vi "Generate 2D scan Waveform.vi"(8 "error in (no error)":errorcluster, 11 "System Parameters [In]":T1={"Optical Parameters"={"Obj. Focal Length [mm]"=0.0, "Scan Lens EFL[mm]"=0.0, "Tube Lens EFL[mm]"=0.0, "Galvo V Range (+/-)"=10.0, "Galvo Max Half Angle [Deg]"=18.0, "Max Galvo Range[%]"=90.0}, "Vibratome"={"Z Bottom [mm]"=0.0, "Pre Cut Dwell [s]"=0.0, "Blade Frequency [RPM]"=0, "Slice Speed [mm/s]"=0.0, "Post Cut Dwell [s]"=0.0, "Ramp Time [s]"=0.0, "Start X [mm]"=0.0, "Start Y [mm]"=0.0, "Slice Length [mm]"=0.0, "Slice Axis"=enum."Y Axis", "Controller VISA Ref"="COM4", "Blade Frequency [Hz]"=0, "Analog Out Channel"="GalvoCtrl/ao0,GalvoCtrl/ao1", "Pixel Clock Source"="/GalvoCtrl/PFI0"}, "Table Stages"={"X Stage"={"Position"=0.0, "Is.Enabled?"=FALSE, "Is.Connected?"=FALSE, "Device SN"="45876539", "AccelerationMaximum"=0.0, "VelocityMaximum"=0.0, "Acceleration"=0.0, "Velocity"=0.0, "waitTimeout (ms)"=0, "Model"=enum."None", "Is.Homed?"=FALSE}, "Y Stage"={"Position"=0.0, "Is.Enabled?"=FALSE, "Is.Connected?"=FALSE, "Device SN"="45876539", "AccelerationMaximum"=0.0, "VelocityMaximum"=0.0, "Acceleration"=0.0, "Velocity"=0.0, "waitTimeout (ms)"=0, "Model"=enum."None", "Is.Homed?"=FALSE}, "Z Stage"={"Position"=0.0, "Is.Enabled?"=FALSE, "Is.Connected?"=FALSE, "Device SN"="45876539", "AccelerationMaximum"=0.0, "VelocityMaximum"=0.0, "Acceleration"=0.0, "Velocity"=0.0, "waitTimeout (ms)"=0, "Model"=enum."None", "Is.Homed?"=FALSE}}, "Imaging Parameter"={"Raster Scan Direction"=enum."Uni Directional", "Pixel Dwell Time [Clock Cycles]"=0, "Flyback Time [Clock Cycles]"=0, "XY Center [um]"={"X"=1.0, "Y"=1.0}, "Pixel Step Size [um] X"=3.0, "XY Image Size"=enum."256 x 256", "Custom"=TRUE, "Custom Size"={"X"=1200, "Y"=1}, "Line Averages"=1, "Pixel Step Size [um] Y"=3.0}, "Galvo HW Parameters"={"Analog Out Channel"="GalvoCtrl/ao0,GalvoCtrl/ao1", "Min Voltage"=-10.0, "Max Voltage"=10.0, "Pixel Clock Source"="/GalvoCtrl/PFI0", "Sample Rate"=1000.0, "Line Clock Out Ch"="GalvoCtrl/port0/line0"}, "Alazar parameters"={"Trigger Settings"={"General Trigger Settings"={"Trigger Operation"=0, "Coupling ID"=2, "Range ID"=2, "Delay"=0, "Timeout Ticks"=0, "Mode"=1, "Parameter"=1}, "Trigger Engine 1"={"Trigger Engine"=0, "Source"=2, "Slope"=1, "Level"=140}, "Trigger Engine 2"={"Trigger Engine"=1000, "Source"=4294967295, "Slope"=1, "Level"=2048}}, "Device ID"={"System ID"=1, "Board ID"=1}, "Ch A Input Control"={"Channel"=1, "Coupling"=2, "Range"=10, "Impedance"=2}, "Ch B Input Control"={"Channel"=2, "Coupling"=2, "Range"=10, "Impedance"=2}, "Acq Settings"={"Record Length"=1440, "Offset"=0, "Records Per Buffer"=2048, "Records Count (Records/Acq)"=2147483647, "Window Type"=1, "Footer"=0, "Samples per record"=2048, "Output Format"=257}, "Capture Clock"={"Sample Rate"=100, "Decimation"=0, "Source"=2, "Edge"=0}}, "Mosaic Paramter"={"X Axis"={"Start [mm]"=0.0, "Steps [pts]"=0.0, "End [mm]"=0.0}, "Y Axis"={"Start [mm]"=0.0, "Steps [pts]"=0.0, "End [mm]"=0.0}, "Scan Pattern"=enum."Uni-directional", "Overlap Options"={"Overlap Type"=enum."No Overlap", "Percent Overlap"=0, "Justify"=enum."Start"}}, "Manual Controls"={"Z0"=10.0, "First image height"=0.0, "Data Path"=path "", "Save parameters"={"start pixel"=45, "#pixels to save"=100}, "Center Galvos"=FALSE, "Acquisition mode"=enum."Alazar FFT", "PSOCT Channel"=1, "Save"=FALSE, "AIP rotation angle"=0.0, "Scan Parameters"={"# Scan"={"#Ascan"=150, "#Bscan"=400}, "# Rpt"={"#ARpt"=1, "#BRpt"=1}, "Aline Rate"=2, "# Extra"={"# ARpt_extra"=5, "#Brtn_extra"=60}}, "ROI Parameters"={"ROI (mm)"={"X (mm)"=1.0, "Y (mm)"=1.0}, "Shift (mm)"={"Xshift (mm)"=0.0, "Yshift (mm)"=0.0}}, "Objective"=30, "ret ds"=FALSE, "Pause?"=FALSE}, "Vibratome Axis"={"Start [mm](first cut height)"=45.85, "slice thickness[um]"=2.1, "#slice"=111, "image thickness(um)"=0.0, "#images"=0, "30um?"=FALSE}} {"Manual Controls"."Objective" items=["5X LKM05", "10X LKM10", "20X LKM20", "10X LSM02"]; "Manual Controls"."Scan Parameters"."Aline Rate" items=["76 KHz", "146 KHz", "76 KHz", "28 KHz", "10 KHz"]; "Manual Controls"."PSOCT Channel" items=["A"=1, "B"=2, "A + B"=3, "C"=4, "A + C"=5, "A + B"=6, "D"=8, "A + D"=9, "B + D"=10, "C + D"=12, "A + B + C + D"=15]; "Alazar parameters"."Capture Clock"."Edge" items=["Rising", "Falling"]; "Alazar parameters"."Capture Clock"."Source" items=["Internal"=1, "Fast External"=2, "Medium External"=3, "Slow External"=4, "External AC"=5, "External DC"=6, "External 10MHz"=7]; "Alazar parameters"."Acq Settings"."Output Format" items=["Float Log"=11, "Float Amp"=10, "U16_LOG"=1, "U16_AMP2"=257, "Real"=3, "Imag"=4]; "Alazar parameters"."Acq Settings"."Footer" items=["FOOTER_NONE", "FOOTER_NPT"]; "Alazar parameters"."Acq Settings"."Window Type" items=["DSP_WINDOW_NONE", "DSP_WINDOW_HANNING", "DSP_WINDOW_HAMMING", "DSP_WINDOW_BLACKMAN", "DSP_WINDOW_BLACKMAN_HARRIS", "DSP_WINDOW_BARTLETT"]; "Alazar parameters"."Ch B Input Control"."Channel" items=["A"=1, "B"=2, "C"=4, "D"=8]; "Alazar parameters"."Ch B Input Control"."Coupling" items=["AC"=1, "DC"=2]; "Alazar parameters"."Ch B Input Control"."Range" items=["20 mV"=1, "40 mV"=2, "50 mV"=3, "80 mV"=4, "100 mV"=5, "200 mV"=6, "400 mV"=7, "500 mV"=8, "800 mV"=9, "1 V"=10, "1.25 V"=33, "2 V"=11, "4 V"=12, "5 V"=13, "8 V"=14, "10 V"=15, "20 V"=16]; "Alazar parameters"."Ch B Input Control"."Impedance" items=["1 MOhm"=1, "50 Ohm"=2, ""=0]; "Alazar parameters"."Ch A Input Control"."Channel" items=["A"=1, "B"=2, "C"=4, "D"=8]; "Alazar parameters"."Ch A Input Control"."Coupling" items=["AC"=1, "DC"=2]; "Alazar parameters"."Ch A Input Control"."Range" items=["20 mV"=1, "40 mV"=2, "50 mV"=3, "80 mV"=4, "100 mV"=5, "200 mV"=6, "400 mV"=7, "500 mV"=8, "800 mV"=9, "1 V"=10, "1.25 V"=33, "2 V"=11, "4 V"=12, "5 V"=13, "8 V"=14, "10 V"=15, "20 V"=16]; "Alazar parameters"."Ch A Input Control"."Impedance" items=["1 MOhm"=1, "50 Ohm"=2, ""=0]; "Alazar parameters"."Trigger Settings"."General Trigger Settings"."Trigger Operation" items=["J", "K", "J OR K", "J AND K", "J XOR K", "J AND NOT K", "NOT J AND K"]; "Alazar parameters"."Trigger Settings"."General Trigger Settings"."Coupling ID" items=["AC"=1, "DC"=2]; "Alazar parameters"."Trigger Settings"."General Trigger Settings"."Range ID" items=["5 V", "1 V", "TTL"]; "Alazar parameters"."Trigger Settings"."Trigger Engine 1"."Trigger Engine" items=["J", "K"]; "Alazar parameters"."Trigger Settings"."Trigger Engine 1"."Source" items=["A", "B", "External", "Disable", "C", "D"]; "Alazar parameters"."Trigger Settings"."Trigger Engine 1"."Slope" items=["Positive"=1, "Negative"=2]; "Alazar parameters"."Trigger Settings"."Trigger Engine 2"."Trigger Engine" items=["J", "K"]; "Alazar parameters"."Trigger Settings"."Trigger Engine 2"."Source" items=["A", "B", "External", "Disable", "C", "D"]; "Alazar parameters"."Trigger Settings"."Trigger Engine 2"."Slope" items=["Positive"=1, "Negative"=2]; "Imaging Parameter"."Pixel Step Size [um] Y" min=0.0 max=10.0 step=0.01; "Imaging Parameter"."Line Averages" min=1 max=30 step=1; "Imaging Parameter"."Flyback Time [Clock Cycles]" max=1000 step=1; "Imaging Parameter"."Pixel Step Size [um] X" min=0.0 max=10.0 step=0.01; "Imaging Parameter"."Custom Size"."Y" min=1 max=30 step=1; "Imaging Parameter"."Custom Size"."X" min=1 max=30 step=1; "Imaging Parameter"."XY Center [um]"."Y" min=1.0 max=30.0 step=1.0; "Imaging Parameter"."XY Center [um]"."X" min=1.0 max=30.0 step=1.0; "Imaging Parameter"."Pixel Dwell Time [Clock Cycles]" max=10 step=1}) -> (0 "error out":errorcluster, 1 "Y":dbl[](graph), 2 "Digital Line Acq":bool[](array[boolean]), 3 "XY":dbl[][](array[numeric]), 5 "X":dbl[](graph), 7 "DO":i16[](graph))   [LabVIEW 2018]
uses:
  Controls/System Parameters.ctl
  Controls/Optical Parameters.ctl
  Controls/Vibratome Parameters.ctl
  Controls/Translation Stage Parameters.ctl
  Hardware Mfg/Thorlabs Translation Stages/Controls/Translation Stage Cluster.ctl
  Controls/Translation Stage Types.ctl
  Controls/Imaging Parameters.ctl
  Controls/Scan Direction.ctl
  type defines/Alazar parameters.ctl
  Hardware Mfg/AlazarTech SDK/Controls/General Trigger Settings.ctl
  Hardware Mfg/AlazarTech SDK/Controls/Trigger Engine Controls.ctl
  Hardware Mfg/AlazarTech SDK/Controls/Alazar Device ID.ctl
  Hardware Mfg/AlazarTech SDK/Controls/Channel Input Controls.ctl
  Hardware Mfg/AlazarTech SDK/Controls/Alazar Acquisition Settings.ctl
  Hardware Mfg/AlazarTech SDK/Controls/Clock Controls.ctl
  type defines/Manual Controls.ctl
  type defines/FFT parameters.ctl
  type defines/FFT mode.ctl
  type defines/Vibratome Param.ctl
panel:
  out "dt":dbl
  # "X"
  # "X"
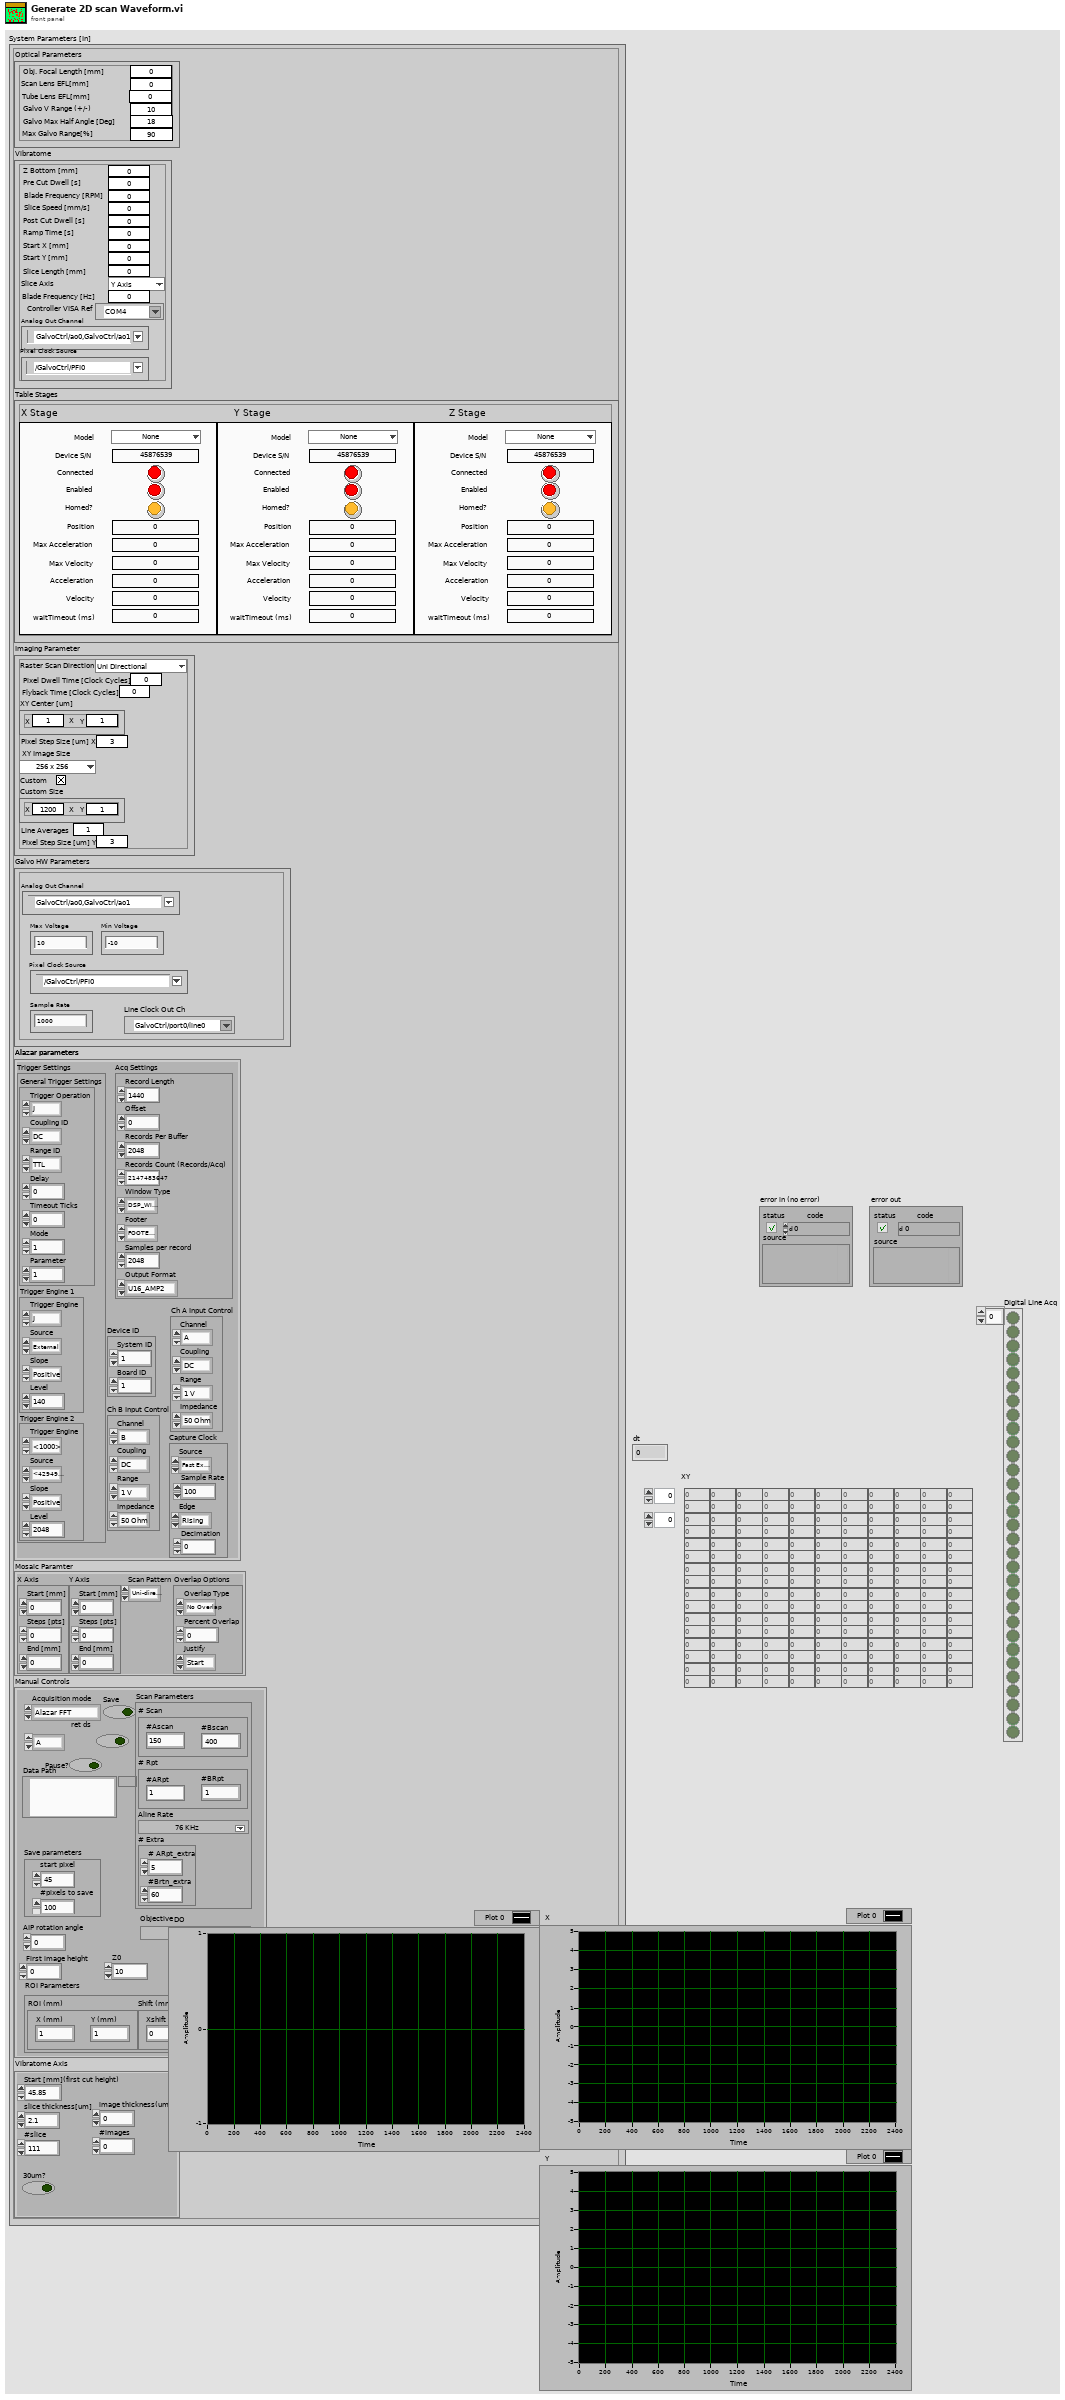
[diagram p1: front panel]
types:
  T1 = typedef "System Parameters.ctl" = cluster{"Optical Parameters":T2, "Vibratome":T3, "Table Stages":T4, "Imaging Parameter":T7, "Galvo HW Parameters":cluster{"Analog Out Channel":tag, "Min Voltage":dbl, "Max Voltage":dbl, "Pixel Clock Source":tag, "Sample Rate":dbl, "Line Clock Out Ch":tag}, "Alazar parameters":T9, "Mosaic Paramter":cluster{"X Axis":cluster{"Start [mm]":dbl, "Steps [pts]":dbl, "End [mm]":dbl}, "Y Axis":cluster{"Start [mm]":dbl, "Steps [pts]":dbl, "End [mm]":dbl}, "Scan Pattern":enum16{"Uni-directional", "Bi-Directional", "Spiral Out", "Spiral In"}, "Overlap Options":cluster{"Overlap Type":enum16{"No Overlap", "X Only", "Y Only", "X and Y"}, "Percent Overlap":u8, "Justify":enum16{"Start", "Center", "End"}}}, "Manual Controls":T16, "Vibratome Axis":T19}
  T2 = typedef "Optical Parameters.ctl" = cluster{"Obj. Focal Length [mm]":dbl, "Scan Lens EFL[mm]":dbl, "Tube Lens EFL[mm]":dbl, "Galvo V Range (+/-)":dbl, "Galvo Max Half Angle [Deg]":dbl, "Max Galvo Range[%]":dbl}
  T3 = typedef "Vibratome Parameters.ctl" = cluster{"Z Bottom [mm]":dbl, "Pre Cut Dwell [s]":dbl, "Blade Frequency [RPM]":u16, "Slice Speed [mm/s]":dbl, "Post Cut Dwell [s]":dbl, "Ramp Time [s]":dbl, "Start X [mm]":dbl, "Start Y [mm]":dbl, "Slice Length [mm]":dbl, "Slice Axis":enum16{"X Axis", "Y Axis", "Z Axis"}, "Controller VISA Ref":refnum<visa-resource-name>, "Blade Frequency [Hz]":u16, "Analog Out Channel":tag, "Pixel Clock Source":tag}
  T4 = typedef "Translation Stage Parameters.ctl" = cluster{"X Stage":T5, "Y Stage":T5, "Z Stage":T5}
  T5 = typedef "Translation Stage Cluster.ctl" = cluster{"Position":dbl, "Is.Enabled?":bool, "Is.Connected?":bool, "Device SN":string, "AccelerationMaximum":dbl, "VelocityMaximum":dbl, "Acceleration":dbl, "Velocity":dbl, "waitTimeout (ms)":i32, "Model":T6, "Is.Homed?":bool}
  T6 = typedef "Translation Stage Types.ctl" = enum16{"None", "Thorlabs LTS", "Thorlabs MLJ"}
  T7 = typedef "Imaging Parameters.ctl" = cluster{"Raster Scan Direction":T8, "Pixel Dwell Time [Clock Cycles]":u16, "Flyback Time [Clock Cycles]":u16, "XY Center [um]":cluster{"X":dbl, "Y":dbl}, "Pixel Step Size [um] X":dbl, "XY Image Size":enum16{"32 x 32", "64 x 64", "128 x 128", "256 x 256", "512 x 512", "1024 x 1024", "2048 x 2048"}, "Custom":bool, "Custom Size":cluster{"X":u16, "Y":u16}, "Line Averages":u8, "Pixel Step Size [um] Y":dbl}
  T8 = typedef "Scan Direction.ctl" = enum16{"Uni Directional", "Bi Directional", "None"}
  T9 = typedef "Alazar parameters.ctl" = cluster{"Trigger Settings":cluster{"General Trigger Settings":T10, "Trigger Engine 1":T11, "Trigger Engine 2":T11}, "Device ID":T12, "Ch A Input Control":T13, "Ch B Input Control":T13, "Acq Settings":T14, "Capture Clock":T15}
  T10 = typedef "General Trigger Settings.ctl" = cluster{"Trigger Operation":u32, "Coupling ID":u32, "Range ID":u32, "Delay":u32, "Timeout Ticks":u32, "Mode":u32, "Parameter":u32}
  T11 = typedef "Trigger Engine Controls.ctl" = cluster{"Trigger Engine":u32, "Source":u32, "Slope":u32, "Level":u32}
  T12 = typedef "Alazar Device ID.ctl" = cluster{"System ID":u32, "Board ID":u32}
  T13 = typedef "Channel Input Controls.ctl" = cluster{"Channel":u8, "Coupling":u32, "Range":u32, "Impedance":u32}
  T14 = typedef "Alazar Acquisition Settings.ctl" = cluster{"Record Length":u32, "Offset":u32, "Records Per Buffer":u32, "Records Count (Records/Acq)":u32, "Window Type":u32, "Footer":u32, "Samples per record":u32, "Output Format":u32}
  T15 = typedef "Clock Controls.ctl" = cluster{"Sample Rate":u32, "Decimation":u32, "Source":u32, "Edge":u32}
  T16 = typedef "Manual Controls.ctl" = cluster{"Z0":dbl, "First image height":dbl, "Data Path":path, "Save parameters":T17, "Center Galvos":bool, "Acquisition mode":T18, "PSOCT Channel":u32, "Save":bool, "AIP rotation angle":dbl, "Scan Parameters":cluster{"# Scan":cluster{"#Ascan":i32, "#Bscan":i32}, "# Rpt":cluster{"#ARpt":i32, "#BRpt":i32}, "Aline Rate":u16, "# Extra":cluster{"# ARpt_extra":i32, "#Brtn_extra":i32}}, "ROI Parameters":cluster{"ROI (mm)":cluster{"X (mm)":dbl, "Y (mm)":dbl}, "Shift (mm)":cluster{"Xshift (mm)":sgl, "Yshift (mm)":sgl}}, "Objective":u16, "ret ds":bool, "Pause?":bool}
  T17 = typedef "FFT parameters.ctl" = cluster{"start pixel":i32, "#pixels to save":i32}
  T18 = typedef "FFT mode.ctl" = enum16{"ThorOCT B line", "ThorOCT Spectral", "ThorOCT FFT", "Alazar B line", "Alazar FFT", "GPU FFT", "Alazar Spectral", "Simulation", "auto adjust focus"}
  T19 = typedef "Vibratome Param.ctl" = cluster{"Start [mm](first cut height)":dbl, "slice thickness[um]":dbl, "#slice":u16, "image thickness(um)":dbl, "#images":u16, "30um?":bool}
  T20 = enum16{"32 x 32", "64 x 64", "128 x 128", "256 x 256", "512 x 512", "1024 x 1024", "2048 x 2048"}
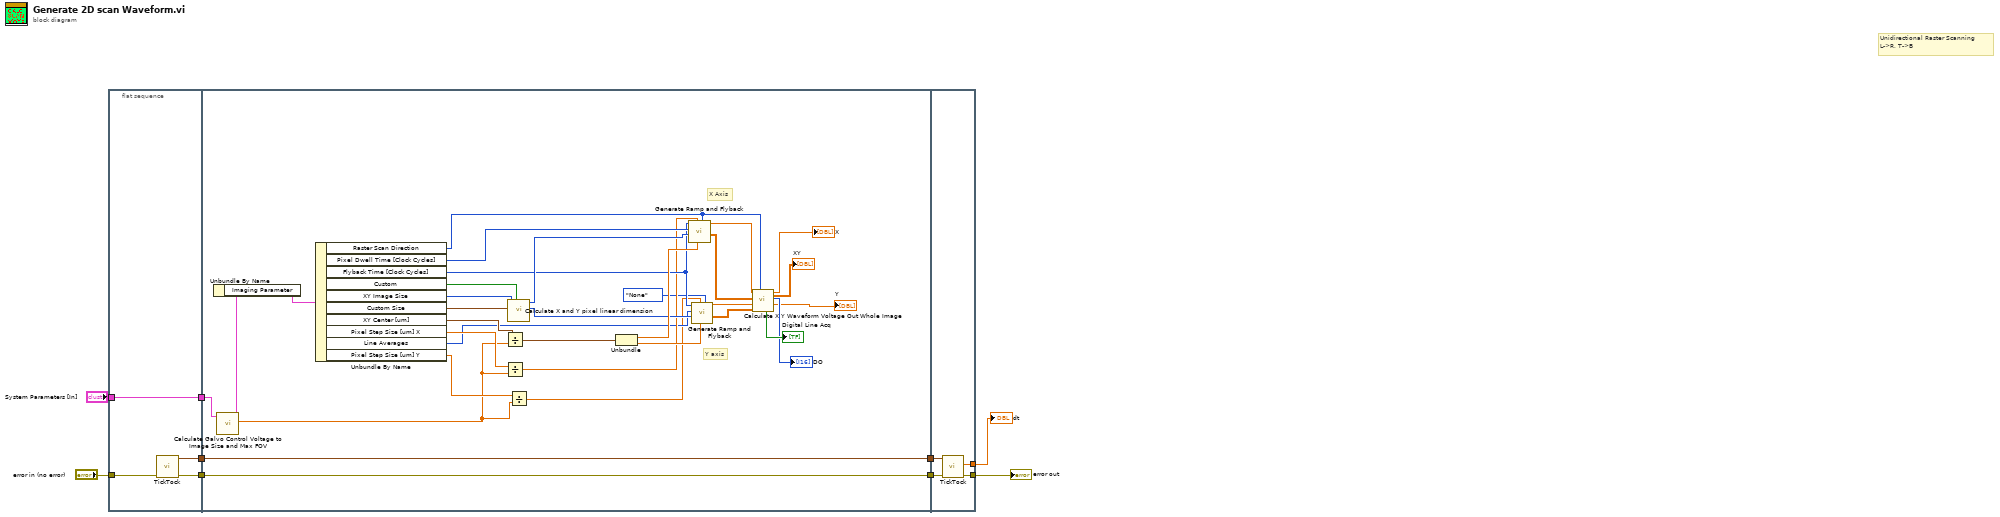
[diagram p0: block diagram]
diagram:
  # "Unidirectional Raster Scanning\nL->R, T->B"
  n1 = flat-sequence {
    tunnel: "System Parameters [In]" -> [w13]
    tunnel: [w13] -> w8
    tunnel: [w12] -> w6
    tunnel: [w11] -> w4
    tunnel: "error in (no error)" -> [w10]
    tunnel: w8 -> [w45]
    tunnel: [w23] -> w7
    tunnel: w6 -> [w23]
    tunnel: [w22] -> w5
    tunnel: w4 -> [w22]
    tunnel: w7 -> [w50]
    tunnel: w5 -> [w49]
    tunnel: [w48] -> w3
    tunnel: [w47] -> w1
    frame #0 {
      n2 = call "TickTock.vi"("Error In"=w10) -> ("Error Out"=w12:errorcluster, "Current Time (Out)"=w11:timestamp)  [unwired: 8 in, 1 out]
    }
    frame #1 {
      # "X Axis"
      # "Y axis"
      n3 = call "Calculate Galvo Control Voltage to Image Size and Max FOV.vi"("System Parameters [In]"=w45) -> ("Galvo [um/V]"=w15:dbl, "System Parameters [Out]"=w44:T1)  [unwired: 7 in, 2 out]
      n4 = Unbundle By Name(w44) -> ("Imaging Parameter"=w46:T7)
      n5 = Unbundle By Name(w46) -> ("Raster Scan Direction"=w24:T8, "Pixel Dwell Time [Clock Cycles]"=w36:u16, "Flyback Time [Clock Cycles]"=w34:u16, "Custom"=w40:bool, "XY Image Size"=w43:T20, "Custom Size"=w42:cluster{"X":u16, "Y":u16}, "XY Center [um]"=w38:cluster{"X":dbl, "Y":dbl}, "Pixel Step Size [um] X"=w39:dbl, "Line Averages"=w30:u8, "Pixel Step Size [um] Y"=w16:dbl)
      n6 = Divide(x=w38, y=w15) -> (x/y=w41:cluster{"X":dbl, "Y":dbl})
      n7 = Divide(x=w39, y=w15) -> (x/y=w31:dbl)
      n8 = call "Calculate X and Y pixel linear dimension.vi"("Imaging Parameter.Custom"=w40, "Custom Size"=w42, "XY Image Resolution"=w43) -> ("Y Px Dim (HFOV)"=w33:u16, "X Px Dim (HFOV)"=w35:u16)  [unwired: 5 in, 2 out]
      n9 = Divide(x=w16, y=w15) -> (x/y=w14:dbl)
      n10 = Unbundle(w41) -> ("X"=w37:dbl, "Y"=w32:dbl)
      n11 = call "Generate Ramp and Flyback.vi"("Raster Scan Direction"=w24, "FOV Center (V)"=w37, "Galvo Step Size Voltages (px/V)"=w31, "Px Dim (HFOV)"=w35, "Pixel Dwell Time [Clock Cycles]"=w36, "Flyback Time [Clock Cycles]"=w34) -> ("Flyback"=w27:dbl[][], "Waveform Graph"=w25:dbl[])  [unwired: 3 in, 1 out]
      n12 = call "Generate Ramp and Flyback.vi"("Raster Scan Direction"=Scan_Direction."None", "FOV Center (V)"=w32, "Galvo Step Size Voltages (px/V)"=w14, "Px Dim (HFOV)"=w33, "Pixel Dwell Time [Clock Cycles]"=w30, "Flyback Time [Clock Cycles]"=w34) -> ("Flyback"=w28:dbl[][], "Waveform Graph"=w26:dbl[])  [unwired: 3 in, 1 out]
      n13 = call "Calculate X Y Waveform Voltage Out Whole Image.vi"("Raster Scan Direction"=w24, "Y Flyback"=w28, "Y Waveform"=w26, "X Flyback"=w27, "X Waveform"=w25) -> ("Y Waveform Out"=→"Y":dbl[], "DO"=→"DO":i16[], "X Waveform Out"=→"X":dbl[], "Digital Line Acq"=→"Digital Line Acq":bool[], "XY Waveform Out"=→"XY":dbl[][])  [unwired: 2 in]
    }
    frame #2 {
      n14 = call "TickTock.vi"("Error In"=w50, "Current Time (In)"=w49) -> ("Error Out"=w47:errorcluster, "dt"=w48:dbl)  [unwired: 7 in, 1 out]
    }
  }
  "dt" <- w3
  "error out" <- w1
